vi "IBM4_Read(IN).vi"(8 "error in":errorcluster, 9 "Number":i32=10, 10 "Channel":i32=3, 11 "COM resource in":refnum<visa-resource-name>="ASRL5::INSTR") -> (0 "error out":errorcluster, 2 "array":i32[](array[numeric]), 3 "COM resource out":refnum<visa-resource-name>="ASRL5::INSTR")   [LabVIEW 2021, in "IBM4.lvlib"]
doc: "This VI interfaces with the IBM4 to perform a read operation.\n\nThe input channel must be between 0 and 3, And the number of readings should be greater than zero. At some point the number of reading will be too high and will cause a timeout error. This should only happen for numbers larger than 10000. The output will be an array of integer values.\n\nAlternate read operations exist covering binary or floating point, single reading, multiple readings, and an average of multiple readings (floating point only)."
uses:
  <instrlib>/IBM4/IBM4.lvlib
panel:
  out "Array":u32[](array[numeric])
  out "read buffer":string="Output 3 = 1.85786 \r\n"
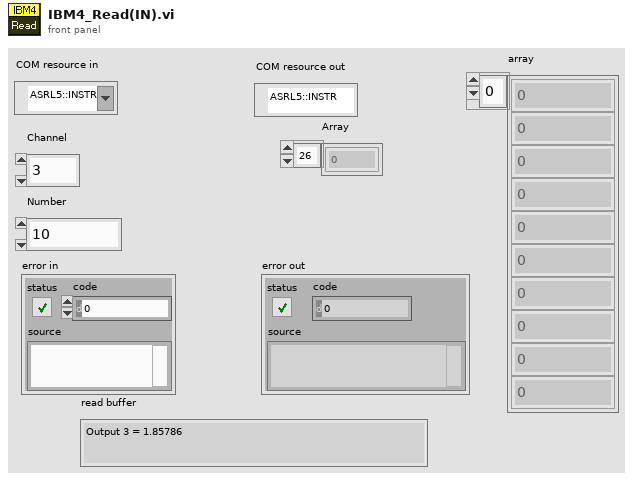
[diagram p1: front panel]
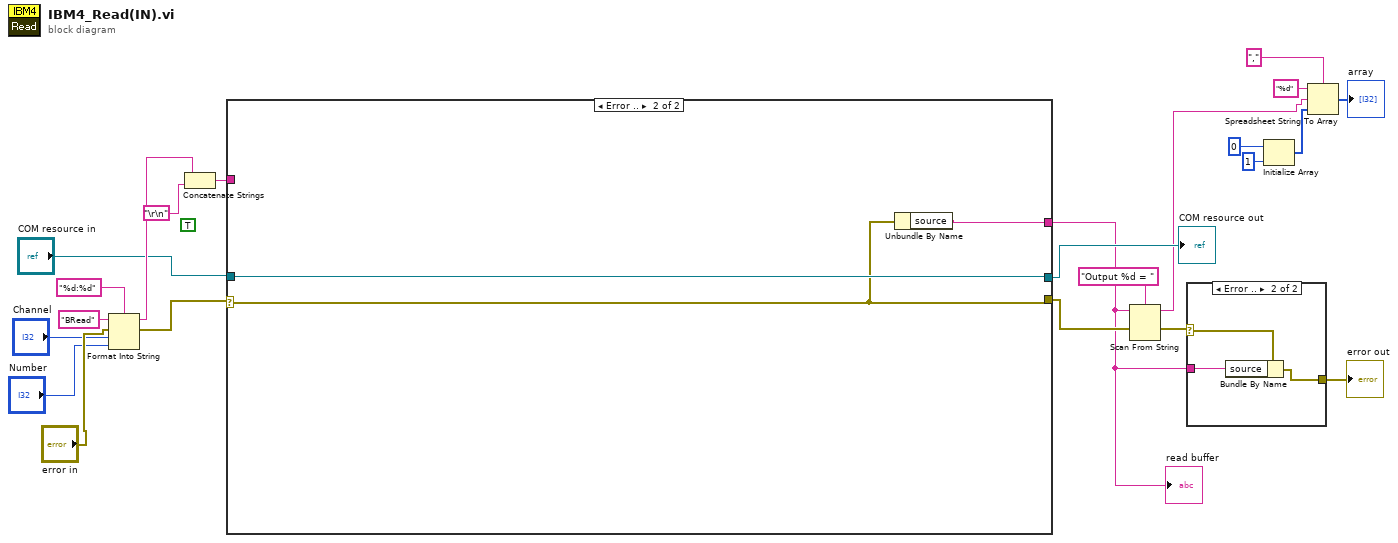
[diagram p0: block diagram]
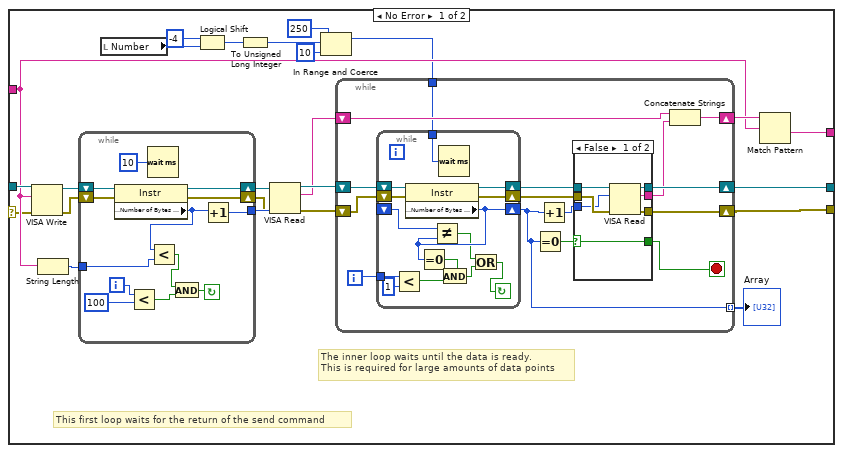
[diagram p3: hidden frame]
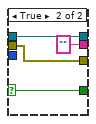
[diagram p4: hidden frame]
diagram:
  (unwired) TRUE ("Enable Termination\nChar (T)")
  n1 = Format Into String(format string="%d:%d", initial string="BRead", error in="error in", "Channel", "Number") -> (resulting string=w14:string, error out=w1:errorcluster)
  n2 = Concatenate Strings(w14, "\r\n") -> (w13:string)
  n3 = case shown="Error .." w1 {
    selector: w1 -> [w34 w101]
    tunnel: "COM resource in" -> [w47 w103]
    tunnel: [w33 w101] -> w17
    tunnel: [w45 w102] -> w10
    tunnel: w13 -> [w44 _]
    tunnel: [w32 w103] -> w18
    frame No Error {
      # "The inner loop waits until the data is ready.\nThis is required for large amounts of data points"
      # "This first loop waits for the return of the send command"
      n4 = VISA Write(VISA resource name=w47, write buffer=w44, error in (no error)=w34) -> (VISA resource name out=w43:refnum<visa-resource-name>, error out=w42:errorcluster)  [unwired: 1 out]
      n5 = String Length(string=w44) -> (length=w35:i32)
      n6 = while {
        tunnel: [w49] -> w40
        shift-right: [w59] -> w41
        shift-left: w43 -> [w60]
        shift-right: [w57] -> w39
        shift-left: w42 -> [w58]
        tunnel: w35 -> [w55]
        i -> [w50]
        stop <- w53 continue-if-true
        n7 = property class="Instr"(reference=w60, error in=w58) -> (reference out=w59:refnum<visa-resource-name>, error out=w57:errorcluster, "Serial Settings:Number of Bytes at Serial Port"=w48:u32)
        n8 = Less?(x=w50, y=100) -> (x < y?=w52:bool)
        n9 = Wait (ms)(milliseconds to wait=u32 10) -> ()  [unwired: 1 out]
        n10 = Less?(x=w48, y=w55) -> (x < y?=w51:bool)
        n11 = And(x=w51, y=w52) -> (x .and. y?=w53:bool)
        n12 = Increment(x=w48) -> (x+1=w49:u32)
      }
      n13 = local read "Number"() -> (w27:i32)
      n14 = Logical Shift(y=i16 -4, x=w27) -> (x << y=w28:i32)
      n15 = To Unsigned Long Integer(number=w28) -> (unsigned 32bit integer=w25:u32)
      n16 = VISA Read(VISA resource name=w41, byte count=w40, error in (no error)=w39) -> (VISA resource name out=w38:refnum<visa-resource-name>, read buffer=w36:string, error out=w37:errorcluster)  [unwired: 1 out]
      n17 = In Range and Coerce(upper limit=u32 250, x=w25, lower limit=u32 10) -> (coerced(x)=w24:u32)  [unwired: 1 out]
      n18 = while {
        shift-right: [w75] -> w32
        shift-left: w38 -> [w73]
        shift-right: [w74] -> w33
        shift-left: w37 -> [w71]
        shift-right: [w69] -> w46
        shift-left: w36 -> [w67]
        tunnel: [w62] -> w31 mode=indexing
        tunnel: w24 -> [w61]
        i -> [w66]
        stop <- w63 stop-if-true
        n19 = while {
          shift-right: [w99] -> w72
          shift-left: w73 -> [w100]
          shift-right: [w97] -> w70
          shift-left: w71 -> [w98]
          tunnel: w66 -> [w96]
          shift-right: [w92] -> w62
          shift-left: _ -> [w91]
          tunnel: w61 -> [w87]
          stop <- w88 continue-if-true
          n20 = Less?(x=w96, y=1) -> (x < y?=w94:bool)
          n21 = property class="Instr"(reference=w100, error in=w98) -> (reference out=w99:refnum<visa-resource-name>, error out=w97:errorcluster, "Serial Settings:Number of Bytes at Serial Port"=w92:u32)
          n22 = Equal To 0?(x=w92) -> (x = 0?=w93:bool)
          n23 = Not Equal?(x=w91, y=w92) -> (x != y?=w89:bool)
          n24 = Wait (ms)(milliseconds to wait=w87) -> ()  [unwired: 1 out]
          n25 = And(x=w93, y=w94) -> (x .and. y?=w90:bool)
          n26 = Or(x=w89, y=w90) -> (x .or. y?=w88:bool)
        }
        n27 = Equal To 0?(x=w62) -> (x = 0?=w64:bool)
        n28 = Increment(x=w62) -> (x+1=w65:u32)
        n29 = case shown="False" w64 {
          selector: w64 -> [w76 w85]
          tunnel: [w82 w86] -> w75
          tunnel: [w81 w84] -> w74
          tunnel: w72 -> [w80 w86]
          tunnel: w70 -> [w79 w84]
          tunnel: [w78 "" ("read buffer")] -> w68
          tunnel: w65 -> [w77 _]
          tunnel: [w76 w85] -> w63
          frame False {
            n30 = VISA Read(VISA resource name=w80, byte count=w77, error in (no error)=w79) -> (VISA resource name out=w82:refnum<visa-resource-name>, read buffer=w78:string, error out=w81:errorcluster)  [unwired: 1 out]
          }
          frame True {
          }
        }
        n31 = Concatenate Strings(w67, w68) -> (w69:string)
      }
      "Array" <- w31
      n32 = Match Pattern(string=w46, regular expression=w44) -> (after substring=w45:string)  [unwired: 1 in, 3 out]
    }
    frame Error {
      n33 = Unbundle By Name(w101) -> ("source"=w102:string)
    }
  }
  "COM resource out" <- w18
  "read buffer" <- w10
  n34 = Scan From String(format string="Output %d = ", input string=w10, error in=w17) -> (remaining string=w4:string, error out=w12:errorcluster)  [unwired: 3 in, 1 out]
  n35 = case shown="Error .." w12 {
    selector: w12 -> [w104 w107]
    tunnel: [w104 w105] -> w11
    tunnel: w10 -> [_ w106]
    frame No Error {
    }
    frame Error {
      n36 = Bundle By Name(cluster=w107, "source"=w106) -> (w105:errorcluster)
    }
  }
  "error out" <- w11
  n37 = Initialize Array(0, 1 ("dimension size")) -> (w8:i32[])
  n38 = Spreadsheet String To Array(delimiter (Tab)=",", format string="%d", spreadsheet string=w4, array type (2D Dbl)=w8) -> (array=→"array":i32[])
